vi "GUNSC_LibCopyImage.vi"(6 "amplifiers":i32, 8 "error in (no error)":errorcluster, 9 "totcols":i32, 10 "bufptr":i32) -> (0 "error out":errorcluster, 2 "return value":i32)   [LabVIEW 2014]
uses:
  public/c/lib/libunsc.so
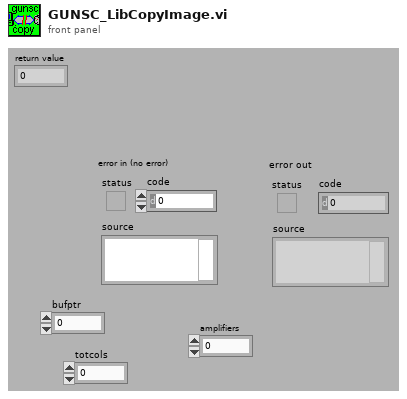
[diagram p1: front panel]
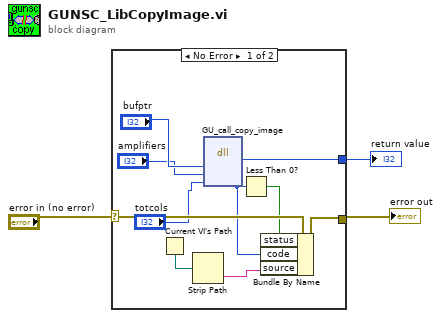
[diagram p0: block diagram]
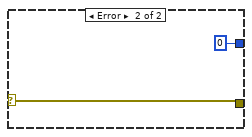
[diagram p2: hidden frame]
diagram:
  n1 = case shown="No Error" "error in (no error)" {
    selector: "error in (no error)" -> [w12 w14]
    tunnel: [w10 0] -> w3
    tunnel: [w7 w14] -> w1
    frame No Error {
      n2 = Current VI's Path() -> (path=w9:path)
      n3 = Strip Path(path=w9) -> (name=w8:string)  [unwired: 1 out]
      n4 = dll-call lib="home/sispi/Panview-1.13.0-64b/PAN/Modules/GUNSC/public/c/lib/libunsc.so" fn="GU_call_copy_image"("buff"="bufptr", "amplifiers"="amplifiers", "totcols"="totcols") -> ("return type"=w10:i32)  [unwired: 6 in, 2 out]
      n5 = Less Than 0?(x=w10) -> (x < 0?=w11:bool)
      n6 = Bundle By Name(cluster=w12, "status"=w11, "code"=w10, "source"=w8) -> (w7:errorcluster)
    }
    frame Error {
    }
  }
  "return value" <- w3
  "error out" <- w1
